vi "Add or Get Virtual Folder.vi"(8 "error in (no error)":errorcluster, 9 "Virtual Folder Name":string, 11 "LVClassLibrary Refnum in":refnum<vi>) -> (0 "error out":errorcluster, 1 "Folder Refnum out":refnum<vi>, 3 "LVClassLibrary Refnum out":refnum<vi>)   [LabVIEW 2021, in "MemberVICreation.lvlib" / "BaseAccessorScripter.lvclass"]
uses:
  <resource>/Framework/Providers/LVClassLibrary/NewAccessors/BaseAccessorScripter/BaseAccessorScripter.lvclass
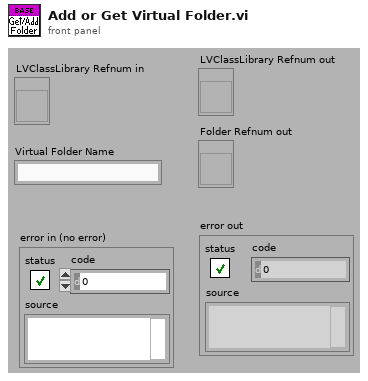
[diagram p1: front panel]
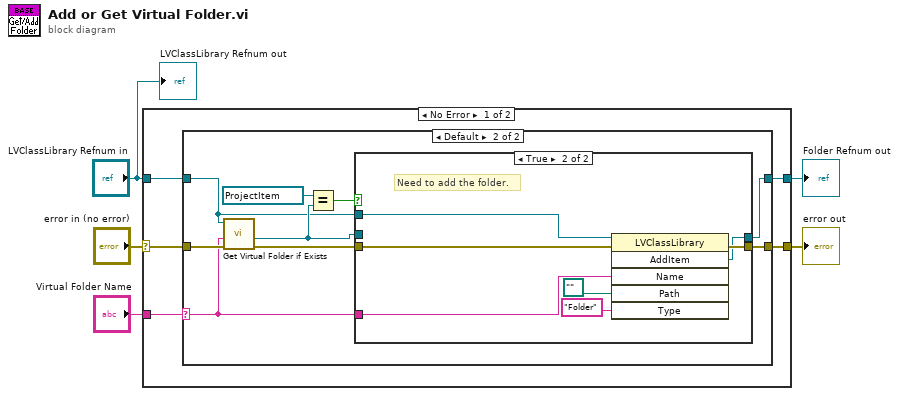
[diagram p0: block diagram]
diagram:
  n1 = case shown="No Error" "error in (no error)" {
    selector: "error in (no error)" -> [w7 w31]
    tunnel: [w6 w31] -> w4
    tunnel: "LVClassLibrary Refnum in" -> [w8 _]
    tunnel: "Virtual Folder Name" -> [w10 _]
    tunnel: [w9 _] -> w1
    frame No Error {
      n2 = case shown="Default" w10 {
        selector: w10 -> [_ w15]
        tunnel: [w12 w17] -> w9
        tunnel: w8 -> [w12 w16]
        tunnel: w7 -> [w11 w21]
        tunnel: [w11 w13] -> w6
        frame "" {
          # "If folder string is empty, just add at the top level (so the folder is the library itself)."
        }
        frame Default {
          n3 = call <resource>:"Get Virtual Folder if Exists.vi"("error in (no error)"=w21, "Virtual Folder Name"=w15, "LVClassLibrary Refnum in"=w16) -> ("error out"=w14:errorcluster, "Folder Refnum out"=w18:refnum<vi>)  [unwired: 7 out]
          n4 = Equal?(x=refnum<vi> refnum ("ProjectItem Refnum"), y=w18) -> (x = y?=w19:bool)
          n5 = case shown="True" w19 {
            tunnel: w18 -> [w23 _]
            tunnel: [w23 w24] -> w17
            tunnel: w16 -> [_ w30]
            tunnel: w15 -> [_ w29]
            tunnel: w14 -> [w22 w27]
            tunnel: [w22 w26] -> w13
            frame False {
              # "Found an existing folder with the requested name."
            }
            frame True {
              # "Need to add the folder."
              n6 = invoke class="LVClassLibrary" method="AddItem"(reference=w30, error in=w27, "Name"=w29, "Path"=path "", "Type"="Folder") -> (error out=w26:errorcluster, "AddItem"=w24:refnum<vi>)  [unwired: 1 in, 4 out]
            }
          }
        }
      }
    }
    frame Error {
    }
  }
  "error out" <- w4
  "Folder Refnum out" <- w1
  "LVClassLibrary Refnum out" <- "LVClassLibrary Refnum in"
